vi "Advanced Fit.vi"(4 "Offset":dbl format="%#_13g", 6 "Sinusoidal Fit Controls.Stat.":T1=enum."Ind. Traces", 8 "error in (no error)":errorcluster, 9 "Response":dbl[][](array[numeric]), 10 "Stimulus":dbl[][](array[numeric]), 11 "Sinusoidal Fit in":refnum<class "Sinusoidal Fit.lvclass">) -> (0 "error out":errorcluster, 2 "Gain and Phase out":T2 {"Phase SD" format="%.1f"; "Phase" format="%.1f"; "Gain SD" format="%.2f"; "Gain" format="%.2f"}, 3 "Sinusoidal Fit out":refnum<class "Sinusoidal Fit.lvclass">)   [LabVIEW 2016, in "Sinusoidal Fit.lvclass"]
uses:
  Sinusoidal Fit.lvclass
  gain and phase/Typedef - Gain and Phase.ctl
  gain and phase/Typedef_StatisticType.ctl
  comm/nan operations/nan operations.lvlib
panel:
  # "Gain:"
  # "+/-"
  # "Phase:"
  # "+/-"
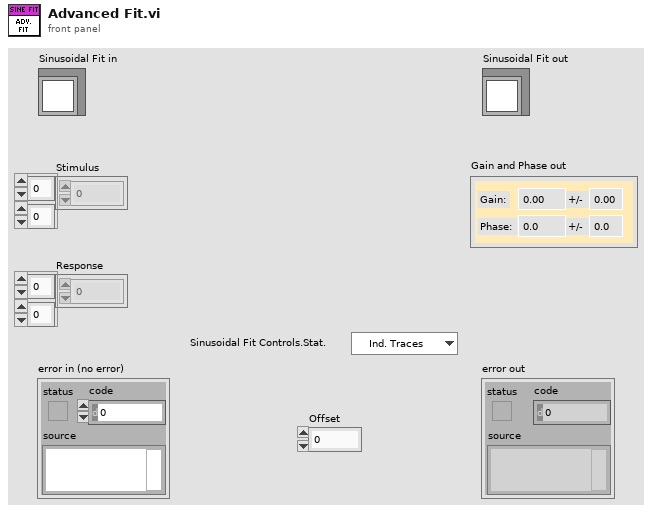
[diagram p1: front panel]
types:
  T1 = typedef "Typedef_StatisticType.ctl" = enum16{"Mean Trace", "Ind. Traces"}
  T2 = typedef "Typedef - Gain and Phase.ctl" = cluster{"Gain":dbl, "Gain SD":dbl, "Phase":dbl, "Phase SD":dbl}
  T3 = typedef "Typedef - Sinusoidal Fit Coefficients.ctl" = cluster{"Offset":dbl, "Gain":dbl, "Phase":dbl, "Freq":dbl}
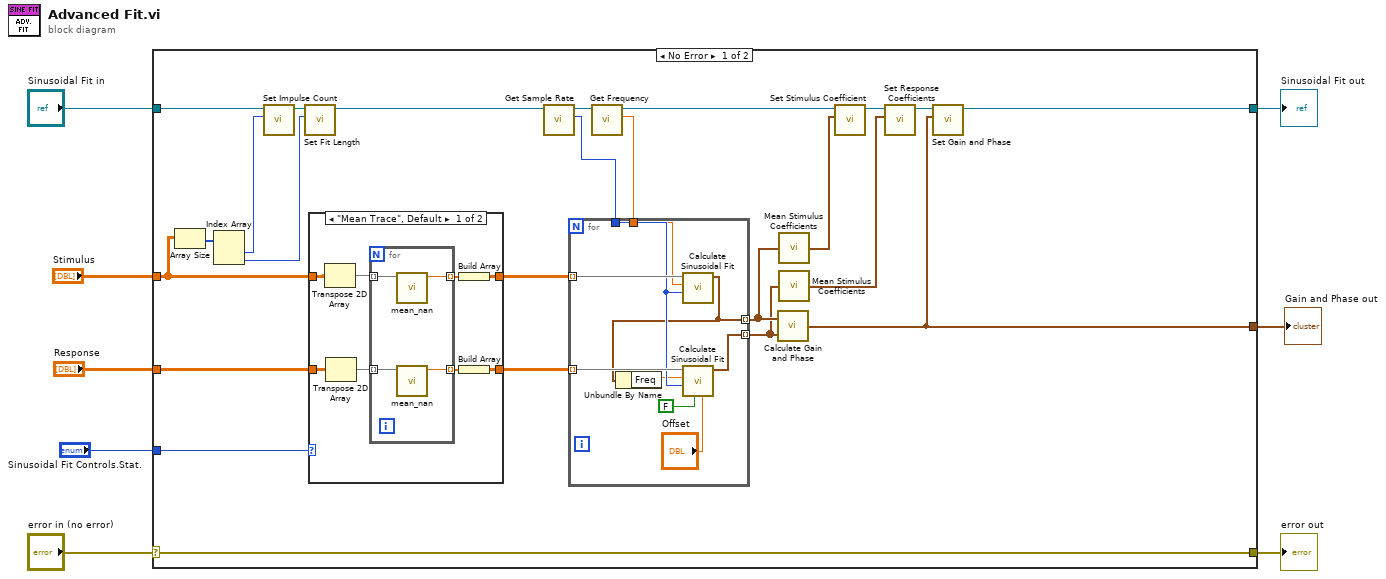
[diagram p0: block diagram]
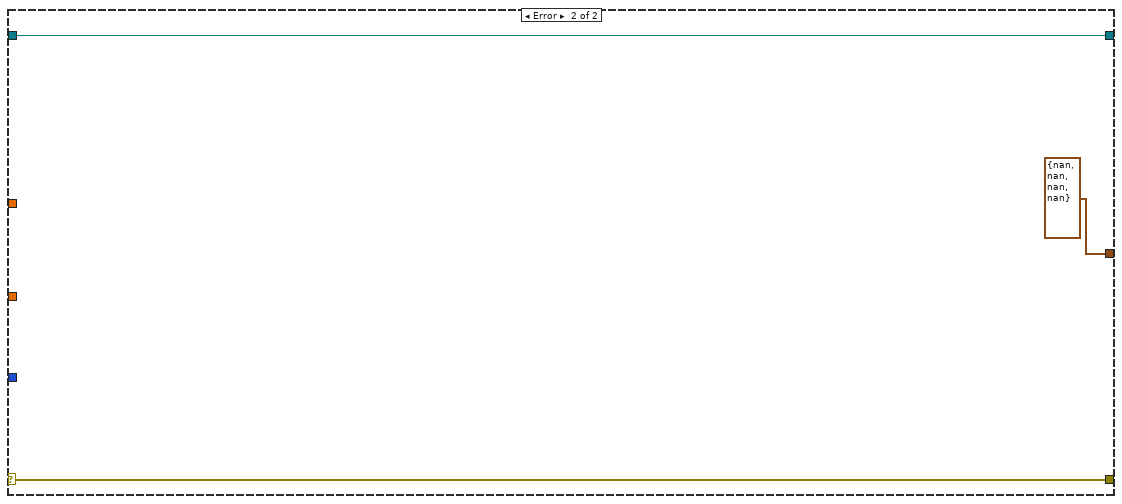
[diagram p3: hidden frame]
diagram:
  n1 = case shown="No Error" "error in (no error)" {
    selector: "error in (no error)" -> [w32 w58]
    tunnel: [w32 w58] -> w7
    tunnel: [w22 w57] -> w5
    tunnel: "Sinusoidal Fit in" -> [w17 w57]
    tunnel: "Stimulus" -> [w27 _]
    tunnel: "Response" -> [w28 _]
    tunnel: [w19 T2 {"Gain"=nan, "Gain SD"=nan, "Phase"=nan, "Phase SD"=nan} ("Gain and Phase out")] -> w2
    tunnel: "Sinusoidal Fit Controls.Stat." -> [w18 _]
    frame No Error {
      n2 = Array Size(array=w27) -> (size(s)=w31:i32[])
      n3 = Index Array(array=w31) -> (element #1=w15:i32, element #2=w14:i32)  [unwired: 2 in]
      n4 = call-dynamic "Set Impulse Count.vi"("Nr of Fit Impulses"=w15, "Abstract Fit in"=w17) -> ("Abstract Fit out"=w16:refnum<class "Sinusoidal Fit.lvclass">)  [unwired: 8 in, 1 out]
      n5 = call-dynamic "Set Fit Length.vi"("Length"=w14, "Abstract Fit in"=w16) -> ("Abstract Fit out"=w13:refnum<class "Sinusoidal Fit.lvclass">)  [unwired: 8 in, 1 out]
      n6 = case shown="\"Mean Trace\", Default" w18 {
        tunnel: [w36 w46] -> w26
        tunnel: [w34 w45] -> w25
        tunnel: w27 -> [w39 w46]
        tunnel: w28 -> [w37 w45]
        frame "Mean Trace", Default {
          n7 = Transpose 2D Array(2D array=w39) -> (transposed array=w40:dbl[][])
          n8 = Transpose 2D Array(2D array=w37) -> (transposed array=w38:dbl[][])
          n9 = for {
            tunnel: [w44] -> w35 mode=indexing
            tunnel: [w43] -> w33 mode=indexing
            tunnel: w40 -> [w42] mode=indexing
            tunnel: w38 -> [w41] mode=indexing
            n10 = call "mean_nan.vi"("Array"=w42) -> ("Mean"=w44:dbl)  [unwired: 10 in]
            n11 = call "mean_nan.vi"("Array"=w41) -> ("Mean"=w43:dbl)  [unwired: 10 in]
          }
          n12 = Build Array(w35) -> (w36:dbl[][])
          n13 = Build Array(w33) -> (w34:dbl[][])
        }
        frame "Ind. Traces" {
        }
      }
      n14 = call-dynamic "Get Sample Rate.vi"("Abstract Fit in"=w13) -> ("Sample Rate"=w12:i32, "Abstract Fit out"=w11:refnum<class "Sinusoidal Fit.lvclass">)  [unwired: 8 in, 1 out]
      n15 = call-dynamic "Get Frequency.vi"("Sinusoidal Fit in"=w11) -> ("Frequency"=w9:dbl, "Sinusoidal Fit out"=w10:refnum<class "Sinusoidal Fit.lvclass">)  [unwired: 8 in, 1 out]
      n16 = for {
        tunnel: [w55] -> w29 mode=indexing
        tunnel: [w51] -> w30 mode=indexing
        tunnel: w26 -> [w54] mode=indexing
        tunnel: w25 -> [w53] mode=indexing
        tunnel: w12 -> [w52]
        tunnel: w9 -> [w50]
        n17 = call "Calculate Sinusoidal Fit.vi"("Sample Rate"=w52, "Stimulus\nFrequency"=w50, "Data in"=w54) -> ("Coefficients"=w51:T3)  [unwired: 7 in, 1 out]
        n18 = Unbundle By Name(w51) -> ("Freq"=w49:dbl)
        n19 = call "Calculate Sinusoidal Fit.vi"("Offset"="Offset", "Ignore Offset"=FALSE, "Sample Rate"=w52, "Stimulus\nFrequency"=w49, "Data in"=w53) -> ("Coefficients"=w55:T3)  [unwired: 5 in, 1 out]
      }
      n20 = call "Calculate Gain and Phase.vi"("Response"=w29, "Stimulus"=w30) -> ("Gain and Phase out"=w19:T2)
      n21 = call "Mean Stimulus Coefficients.vi"("Coefficients in"=w30) -> ("Mean Coefficients out"=w21:T3)
      n22 = call "Mean Stimulus Coefficients.vi"("Coefficients in"=w29) -> ("Mean Coefficients out"=w20:T3)
      n23 = call-dynamic "Set Stimulus Coefficient.vi"("Coefficients"=w21, "Sinusoidal Fit in"=w10) -> ("Sinusoidal Fit out"=w23:refnum<class "Sinusoidal Fit.lvclass">)  [unwired: 8 in, 1 out]
      n24 = call-dynamic "Set Response Coefficients.vi"("Coefficients"=w20, "Sinusoidal Fit in"=w23) -> ("Sinusoidal Fit out"=w24:refnum<class "Sinusoidal Fit.lvclass">)  [unwired: 8 in, 1 out]
      n25 = call-dynamic "Set Gain and Phase.vi"("Gain and Phase"=w19, "Sinusoidal Fit in"=w24) -> ("Sinusoidal Fit out"=w22:refnum<class "Sinusoidal Fit.lvclass">)  [unwired: 8 in, 1 out]
    }
    frame Error {
    }
  }
  "error out" <- w7
  "Sinusoidal Fit out" <- w5
  "Gain and Phase out" <- w2
